vi "GetData.vi"   [LabVIEW 2017]
uses:
  <vilib>/Utility/file.llb/Read Delimited Spreadsheet (string).vi
types:
  T1 = enum16{"open", "replace", "create", "open or create", "replace or create", "replace or create with confirmation"}
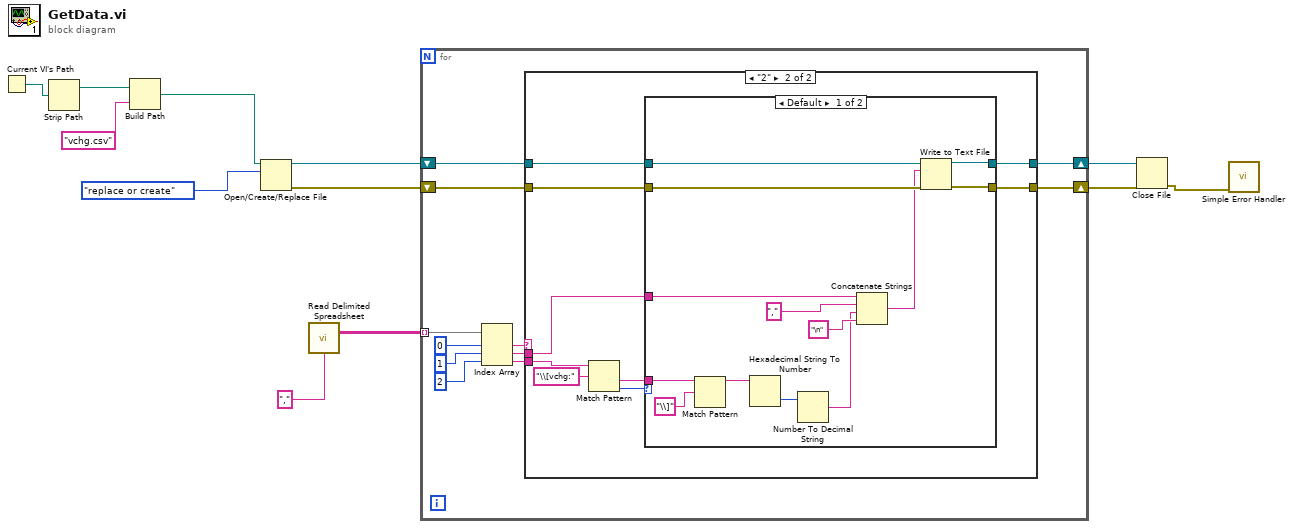
[diagram p0: block diagram]
diagram:
  n1 = Current VI's Path() -> (path=w10:path)
  n2 = Strip Path(path=w10) -> (stripped path=w9:path)  [unwired: 1 out]
  n3 = Build Path(base path=w9, name or relative path="vchg.csv") -> (appended path=w7:path)
  n4 = Open/Create/Replace File(file path (use dialog)=w7, operation (0:open)=T1."replace or create") -> (refnum out=w6:refnum<file>, error out=w5:errorcluster)  [unwired: 4 in, 1 out]
  n5 = call-poly <vilib>:"Read Delimited Spreadsheet.vi"("delimiter (\\t)"="," ("delimiter (\\t)")) -> ("all rows"=w11:string[][])  [unwired: 9 in, 5 out]
  n6 = for {
    tunnel: w11 -> [w23] mode=indexing
    shift-right: [w17] -> w4
    shift-left: w6 -> [w19]
    shift-right: [w16] -> w3
    shift-left: w5 -> [w18]
    n7 = Index Array(array=w23, index #1=0 ("index"), index #2=1 ("index"), index #3=2 ("index")) -> (element #1=w13:string, element #2=w15:string, element #3=w14:string)
    n8 = case shown="\"2\"" w13 {
      tunnel: w19 -> [w25 w32]
      tunnel: w18 -> [w24 w31]
      tunnel: [w25 w28] -> w17
      tunnel: [w24 w29] -> w16
      tunnel: w15 -> [_ w27]
      tunnel: w14 -> [_ w34]
      frame Default {
      }
      frame "2" {
        n9 = Match Pattern(string=w34, regular expression="\\[vchg:") -> (after substring=w26:string, offset past match=w30:i32)  [unwired: 1 in, 2 out]
        n10 = case shown="Default" w30 {
          tunnel: w32 -> [w44 w49]
          tunnel: w31 -> [w43 w48]
          tunnel: [w41 w48] -> w29
          tunnel: [w42 w49] -> w28
          tunnel: w26 -> [w39 _]
          tunnel: w27 -> [w47 _]
          frame Default {
            n11 = Match Pattern(string=w39, regular expression="\\]") -> (before substring=w37:string)  [unwired: 1 in, 3 out]
            n12 = Hexadecimal String To Number(string=w37) -> (number=w36:u32)  [unwired: 2 in, 1 out]
            n13 = Number To Decimal String(number=w36) -> (decimal integer string=w35:string)  [unwired: 1 in]
            n14 = Concatenate Strings(w47, "," ("string"), w35, "\n" ("string")) -> (w40:string)
            n15 = Write to Text File(file (use dialog)=w44, text=w40, error in=w43) -> (refnum out=w42:refnum<file>, error out=w41:errorcluster)  [unwired: 1 in, 1 out]
          }
          frame ..-1 {
          }
        }
      }
    }
  }
  n16 = Close File(refnum=w4, error in=w3) -> (error out=w1:errorcluster)  [unwired: 1 out]
  n17 = call <vilib>:"Simple Error Handler.vi"("error in (no error)"=w1) -> ()  [unwired: 4 in, 5 out]
